vi "sensor2.vi"(3 "Sensor":string) -> (0 "1":bool, 1 "2":bool)   [LabVIEW 2023]
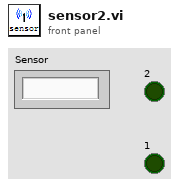
[diagram p1: front panel]
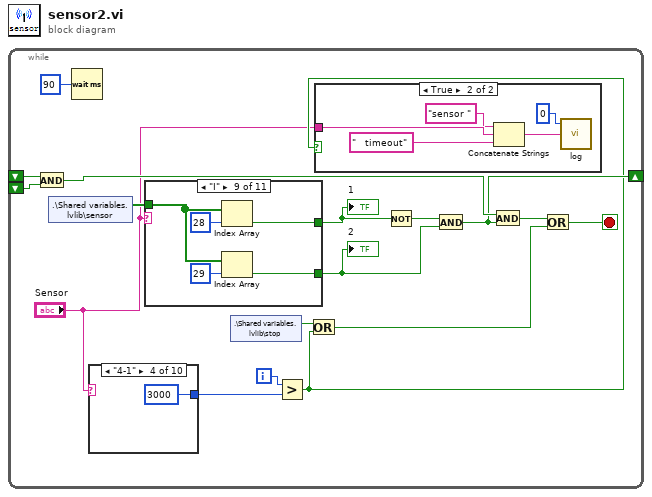
[diagram p0: block diagram]
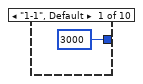
[diagram p3: hidden frame]
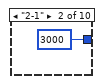
[diagram p4: hidden frame]
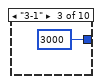
[diagram p5: hidden frame]
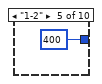
[diagram p6: hidden frame]
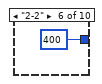
[diagram p7: hidden frame]
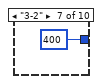
[diagram p8: hidden frame]
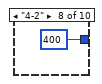
[diagram p9: hidden frame]
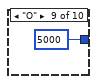
[diagram p10: hidden frame]
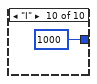
[diagram p11: hidden frame]
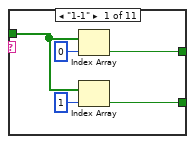
[diagram p12: hidden frame]
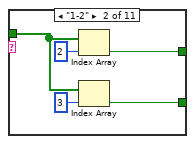
[diagram p13: hidden frame]
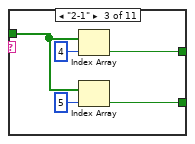
[diagram p14: hidden frame]
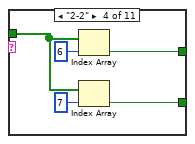
[diagram p15: hidden frame]
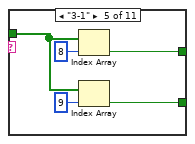
[diagram p16: hidden frame]
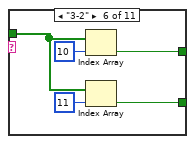
[diagram p17: hidden frame]
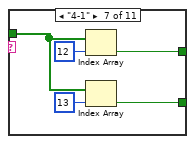
[diagram p18: hidden frame]
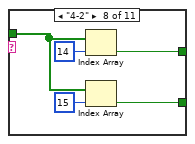
[diagram p19: hidden frame]
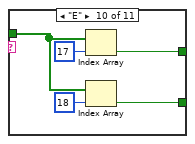
[diagram p20: hidden frame]
diagram:
  n1 = while {
    shift-right: [w13] -> _
    shift-left: _ -> [w16]
    shift-left: _ -> [w15]
    i -> [w4]
    stop <- w7 stop-if-true
    n2 = And(x=w16, y=w15) -> (x .and. y?=w14:bool)
    n3 = shared-variable ".\\Shared variables.lvlib\\sensor"() -> (w9:bool[])  [unwired: 1 in, 1 out]
    n4 = Wait (ms)(milliseconds to wait=u32 90) -> ()  [unwired: 1 out]
    n5 = case shown="\"4-1\"" "Sensor" {
      tunnel: [3000 ("y") 3000 ("y") 3000 ("y") 3000 ("y") 400 ("y") 400 ("y") 400 ("y") 400 ("y") 5000 ("y") 1000 ("y")] -> w3
      frame "1-1", Default {
      }
      frame "2-1" {
      }
      frame "3-1" {
      }
      frame "4-1" {
      }
      frame "1-2" {
      }
      frame "2-2" {
      }
      frame "3-2" {
      }
      frame "4-2" {
      }
      frame "O" {
      }
      frame "I" {
      }
    }
    n6 = case shown="\"I\"" "Sensor" {
      tunnel: [w36 w40 w45 w50 w55 w60 w65 w70 w74 w79 w84] -> w11
      tunnel: [w34 w39 w44 w49 w54 w59 w64 w69 w73 w78 w83] -> w10
      tunnel: w9 -> [w33 w38 w43 w48 w53 w58 w63 w68 w75 w80 w85]
      frame "1-1" {
        n7 = Index Array(array=w33, index=0) -> (element=w36:bool)
        n8 = Index Array(array=w33, index=1) -> (element=w34:bool)
      }
      frame "1-2" {
        n9 = Index Array(array=w38, index=2) -> (element=w40:bool)
        n10 = Index Array(array=w38, index=3) -> (element=w39:bool)
      }
      frame "2-1" {
        n11 = Index Array(array=w43, index=4) -> (element=w45:bool)
        n12 = Index Array(array=w43, index=5) -> (element=w44:bool)
      }
      frame "2-2" {
        n13 = Index Array(array=w48, index=6) -> (element=w50:bool)
        n14 = Index Array(array=w48, index=7) -> (element=w49:bool)
      }
      frame "3-1" {
        n15 = Index Array(array=w53, index=8) -> (element=w55:bool)
        n16 = Index Array(array=w53, index=9) -> (element=w54:bool)
      }
      frame "3-2" {
        n17 = Index Array(array=w58, index=10) -> (element=w60:bool)
        n18 = Index Array(array=w58, index=11) -> (element=w59:bool)
      }
      frame "4-1" {
        n19 = Index Array(array=w63, index=12) -> (element=w65:bool)
        n20 = Index Array(array=w63, index=13) -> (element=w64:bool)
      }
      frame "4-2" {
        n21 = Index Array(array=w68, index=14) -> (element=w70:bool)
        n22 = Index Array(array=w68, index=15) -> (element=w69:bool)
      }
      frame "I" {
        n23 = Index Array(array=w75, index=28) -> (element=w74:bool)
        n24 = Index Array(array=w75, index=29) -> (element=w73:bool)
      }
      frame "E" {
        n25 = Index Array(array=w80, index=17) -> (element=w79:bool)
        n26 = Index Array(array=w80, index=18) -> (element=w78:bool)
      }
      frame "O", Default {
        n27 = Index Array(array=w85, index=30) -> (element=w84:bool)
        n28 = Index Array(array=w85, index=31) -> (element=w83:bool)
      }
    }
    "2" <- w10
    "1" <- w11
    n29 = shared-variable ".\\Shared variables.lvlib\\stop"() -> (w6:bool)  [unwired: 1 in, 1 out]
    n30 = Greater?(x=w4, y=w3) -> (0:w2:bool)
    n31 = Or(x=w6, y=w2) -> (x .or. y?=w5:bool)
    n32 = case shown="True" w2 {
      tunnel: "Sensor" -> [_ w22]
      frame False {
      }
      frame True {
        n33 = Concatenate Strings("sensor " ("string"), w22, "   timeout" ("string")) -> (w19:string)
        n34 = call "log.vi"("worker"=i8 0, "input string"=w19) -> ()  [unwired: 6 in, 3 out]
      }
    }
    n35 = Not(x=w11) -> (.not. x?=w17:bool)
    n36 = And(x=w17, y=w10) -> (x .and. y?=w13:bool)
    n37 = And(x=w14, y=w13) -> (x .and. y?=w8:bool)
    n38 = Or(x=w8, y=w5) -> (x .or. y?=w7:bool)
  }
